vi "Configure Hardware.vi"(8 "error in (no error)":errorcluster caption="错误输入（无错误）", 11 "Hardware Resources in":T1 caption="硬件资源输入") -> (0 "error out":errorcluster caption="错误输出", 3 "Hardware Resources out":T1 caption="硬件资源输出")   [LabVIEW 2014, in "Acquisition.lvlib"]
doc: "配置硬件。"
uses:
  Acquisition.lvlib
  Hardware Configuration.ctl
  <vilib>/DAQmx/create/channels.llb/DAQmx Create Channel (AI-Voltage-Basic).vi
  <vilib>/DAQmx/configure/timing.llb/DAQmx Timing (Sample Clock).vi
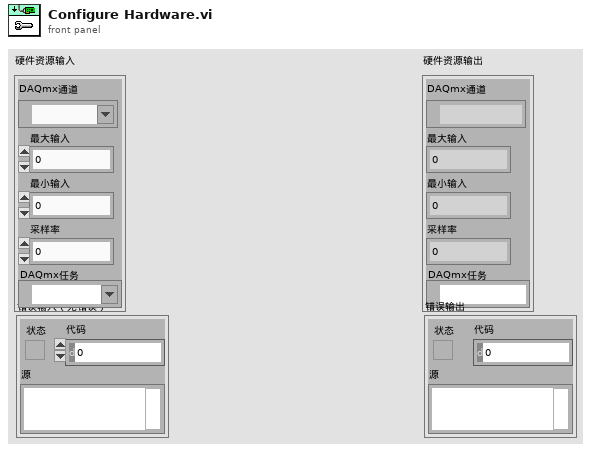
[diagram p1: front panel]
types:
  T1 = typedef "Acquisition.lvlib/Hardware Configuration.ctl" = cluster{"DAQmx Channel":tag, "Max Input":dbl, "Min Input":dbl, "Sample Rate":dbl, "DAQmx Task":refnum<k21>}
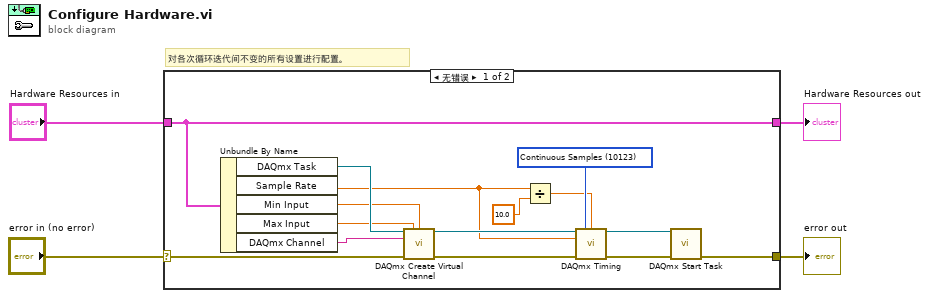
[diagram p0: block diagram]
diagram:
  # "对各次循环迭代间不变的所有设置进行配置。"
  n1 = case shown="无错误" "error in (no error)" {
    selector: "error in (no error)" -> [w13 w20]
    tunnel: [w5 w20] -> w3
    tunnel: "Hardware Resources in" -> [w12 w21]
    tunnel: [w12 w21] -> w1
    frame No Error {
      w11 = 10123 items=["Finite Samples"=10178, "Continuous Samples"=10123, "Hardware Timed Single Point"=12522] ("sample mode")
      n2 = Unbundle By Name(w12) -> ("DAQmx Task"=w19:refnum<k21>, "Sample Rate"=w10:dbl, "Min Input"=w16:dbl, "Max Input"=w17:dbl, "DAQmx Channel"=w18:tag)
      n3 = call-poly <vilib>:"DAQmx Create Virtual Channel.vi"("task in"=w19, "maximum value"=w17, "minimum value"=w16, "physical channels"=w18, "error in"=w13) -> ("task out"=w15:refnum<k21>, "error out"=w14:errorcluster)  [unwired: 9 in]
      n4 = Divide(x=w10, y=10.0) -> (x/y=w8:dbl)
      n5 = call-poly <vilib>:"DAQmx Timing.vi"("task/channels in"=w15, "sample mode"=w11, "samples per channel"=w8, "rate"=w10, "error in"=w14) -> ("task out"=w6:refnum<k21>, "error out"=w7:errorcluster)  [unwired: 9 in]
      n6 = call <vilib>:"DAQmx Start Task.vi"("task/channels in"=w6, "error in"=w7) -> ("error out"=w5:errorcluster)  [unwired: 12 in, 1 out]
    }
    frame Error {
    }
  }
  "Hardware Resources out" <- w1
  "error out" <- w3
